vi "RPC Method Greeter SayHello.vi"(8 "error in (no error)":errorcluster, 11 "OOP Server in":refnum<class "Greeter.lvclass">) -> (0 "error out":errorcluster, 3 "OOP Server out":refnum<class "Greeter.lvclass">)   [LabVIEW 2019, in "helloworld_server.lvlib" / "Greeter.lvclass"]
uses:
  Greeter.lvclass
  Greeter.lvclass/Greeter.ctl
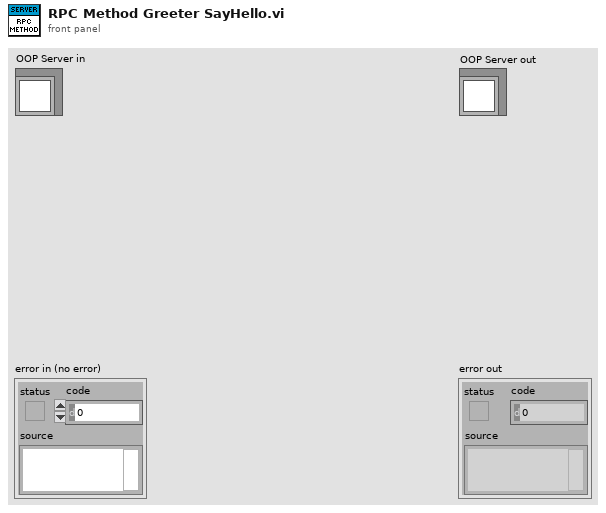
[diagram p1: front panel]
types:
  T1 = typedef "helloworld_server.lvlib/Greeter.lvclass/Server Internal UEs.ctl" = cluster{"Greeter SayHello Internal UE":refnum<user-event>}
  T2 = typedef "helloworld_server.lvlib/Greeter.lvclass/Server gRPC UEs.ctl" = cluster{"Greeter SayHello gRPC UE":refnum<user-event>}
  T3 = typedef "grpc-lvsupport-release.lvlib/grpcId.ctl" = u64
  T4 = typedef "helloworld_server.lvlib/helloworld_HelloRequest.ctl" = cluster{"name":string}
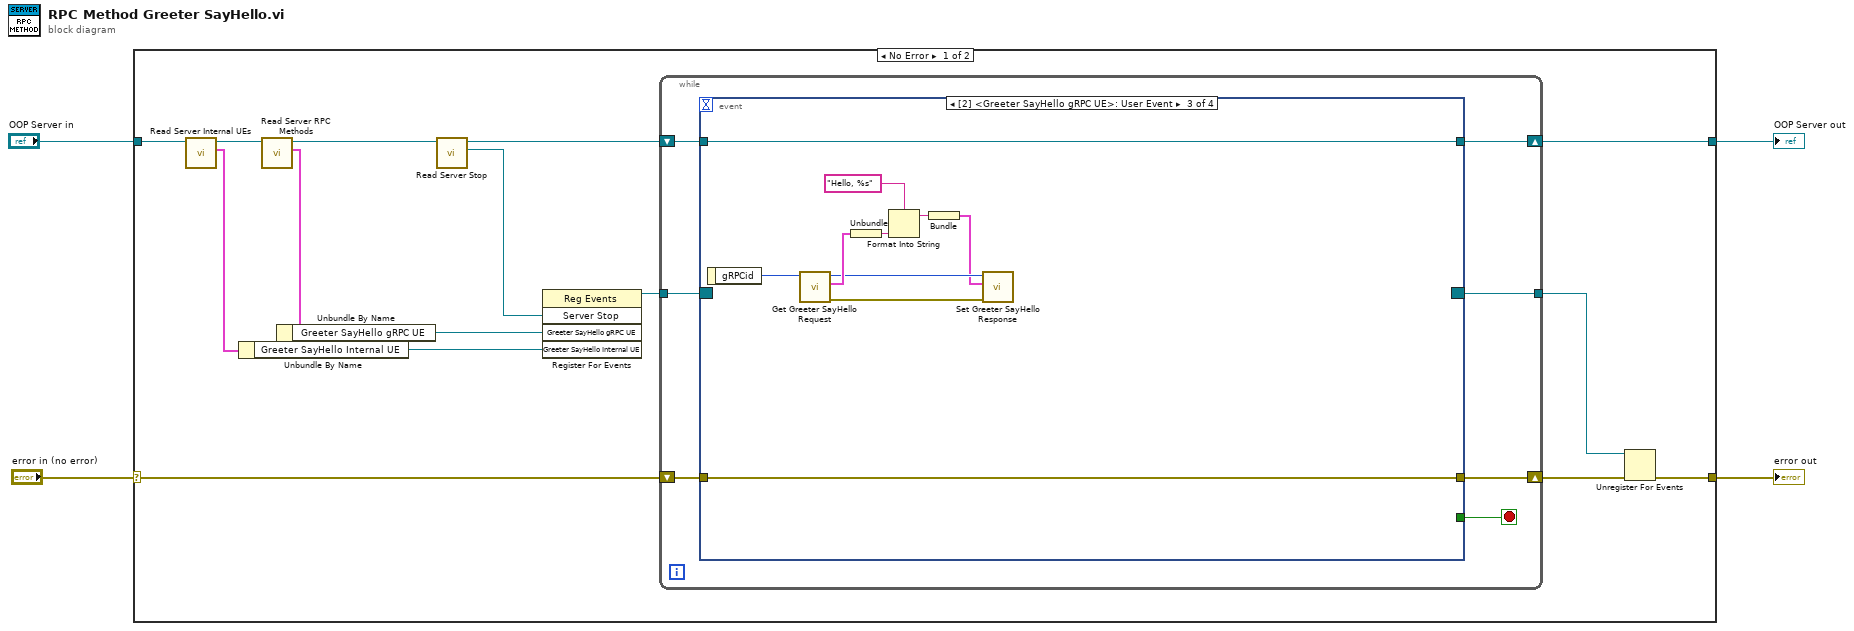
[diagram p0: block diagram]
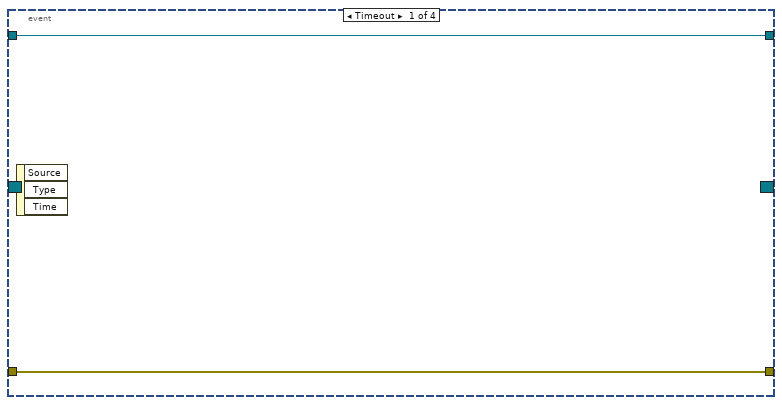
[diagram p2: hidden frame]
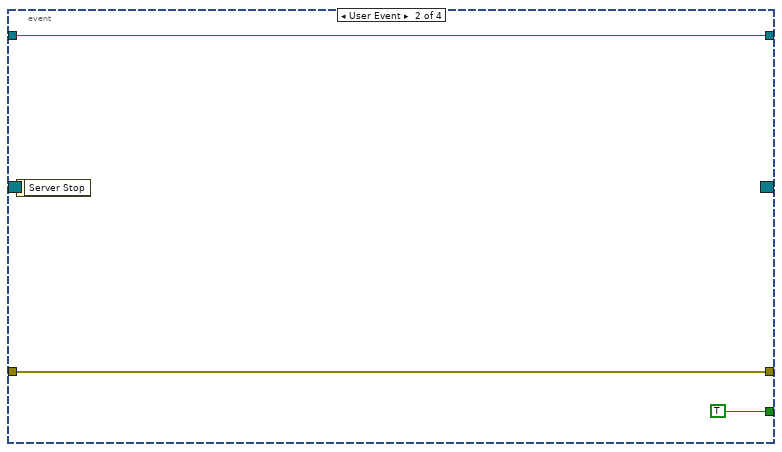
[diagram p3: hidden frame]
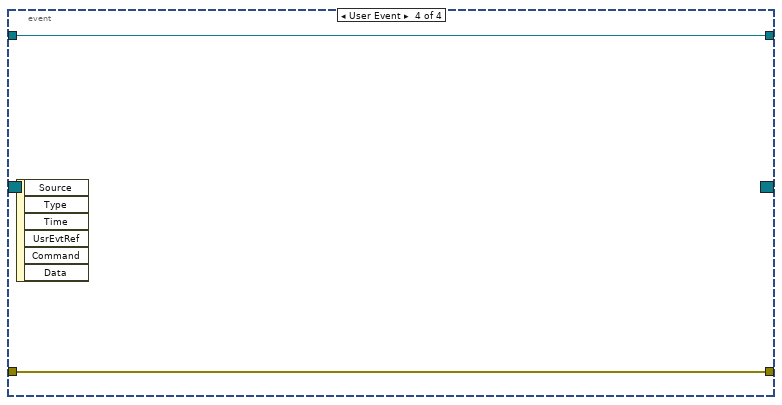
[diagram p4: hidden frame]
diagram:
  n1 = case shown="No Error" "error in (no error)" {
    selector: "error in (no error)" -> [w15 w45]
    tunnel: [w13 w45] -> w3
    tunnel: "OOP Server in" -> [w17 w44]
    tunnel: [w5 w44] -> w1
    frame No Error {
      n2 = call "Read Server Internal UEs.vi"("SignalGeneratorService in"=w17) -> ("Server Internal UEs"=w9:T1, "SignalGeneratorService out"=w16:refnum<class "Greeter.lvclass">)  [unwired: 8 in, 1 out]
      n3 = Unbundle By Name ("Unbundle Internal UE")(w9) -> ("Greeter SayHello Internal UE"=w8:refnum<user-event>)
      n4 = call "Read Server RPC Methods.vi"("SignalGeneratorService in"=w16) -> ("Server RPC Methods"=w11:T2, "SignalGeneratorService out"=w6:refnum<class "Greeter.lvclass">)  [unwired: 8 in, 1 out]
      n5 = Unbundle By Name ("Unbundle gRPC UE")(w11) -> ("Greeter SayHello gRPC UE"=w10:refnum<user-event>)
      n6 = call-dynamic "Read Server Stop.vi"("iService in"=w6) -> ("Server Stop"=w19:refnum<user-event>, "iService out"=w7:refnum<class "Greeter.lvclass">)  [unwired: 8 in, 1 out]
      n7 = register-events(w19, w10, w8) -> (reference out=w18:refnum<event-registration>)  [unwired: 2 in, 1 out]
      n8 = while {
        tunnel: w18 -> [w26]
        tunnel: [w22] -> w12
        shift-right: [w23] -> w14
        shift-left: w15 -> [w24]
        shift-right: [w20] -> w5
        shift-left: w7 -> [w21]
        stop <- w25 stop-if-true
        n9 = event "RPC Method Event Structure" shown="[2] <Greeter SayHello gRPC UE>: User Event" {
          selector: w26 -> [_ _ _ _]
          dyn-events: [_ _ _ _] -> w22
          timeout: _ -> [_ _ _ _]
          tunnel: [_ TRUE _ _] -> w25
          tunnel: w24 -> [w28 w30 w41 w43]
          tunnel: [w28 w30 w41 w43] -> w23
          tunnel: w21 -> [w27 w29 w40 w42]
          tunnel: [w27 w29 w40 w42] -> w20
          event Timeout {
            n10 = event-data() -> ()  [unwired: 1 in, 3 out]
          }
          event User Event {
            n11 = event-data() -> ()  [unwired: 1 in, 1 out]
          }
          event User Event {
            n12 = event-data() -> ("gRPCid"=w32:T3)  [unwired: 1 in]
            n13 = call "Get Greeter SayHello Request.vi"("gRPCid"=w32) -> ("error out"=w34:errorcluster, "Message Data"=w36:T4, "gRPCid out"=w35:T3)  [unwired: 8 in]
            n14 = Unbundle(w36) -> ("name"=w39:string)
            n15 = Format Into String(format string="Hello, %s", w39) -> (resulting string=w37:string)  [unwired: 2 in, 1 out]
            n16 = Bundle(w37) -> (w33:cluster{string})  [unwired: 1 in]
            n17 = call "Set Greeter SayHello Response.vi"("error in (no error)"=w34, "Message Data"=w33, "gRPCid in"=w35) -> ()  [unwired: 8 in, 1 out]
          }
          event User Event {
            n18 = event-data() -> ()  [unwired: 1 in, 6 out]
          }
        }
      }
      n19 = Unregister For Events(event registration refnum=w12, error in=w14) -> (error out=w13:errorcluster)
    }
    frame Error {
    }
  }
  "error out" <- w3
  "OOP Server out" <- w1
